vi "Resize.vi"(8 "error in (no error)":errorcluster, 10 "Pane.Content Area Rect":T1, 11 "Loop data in":T2 {"PanelMap"."Data"."Plot Bounds (%)"."Bottom (%)" format="%.2f"; "PanelMap"."Data"."Plot Bounds (%)"."Top (%)" format="%.2f"; "PanelMap"."Data"."Plot Bounds (%)"."Right (%)" format="%.2f"; "PanelMap"."Data"."Plot Bounds (%)"."Left (%)" format="%.2f"}) -> (0 "error out":errorcluster, 3 "Loop data out":T2 {"PanelMap"."Data"."Plot Bounds (%)"."Bottom (%)" format="%.2f"; "PanelMap"."Data"."Plot Bounds (%)"."Top (%)" format="%.2f"; "PanelMap"."Data"."Plot Bounds (%)"."Right (%)" format="%.2f"; "PanelMap"."Data"."Plot Bounds (%)"."Left (%)" format="%.2f"})   [LabVIEW 2021, in "MultiStokePlot.lvlib" / "MultiPlotPanel.lvclass"]
uses:
  Classes/MultiPlotPanel/MultiPlotPanel.lvclass
  Loop Data.ctl
  <vilib>/IlluminatedG/IG OOPanel/OOPanel/Manager/Manager.lvclass
  Panel Map.ctl
  Panel Map Data.ctl
  <userlib>/bjustice/RocketPlot/Classes/RocketPlotPanel/RocketPlotPanel.lvclass
  Window Position.ctl
  <vilib>/IlluminatedG/IG OOPanel/OOPanel/Panel/Panel Events.ctl
  <vilib>/IlluminatedG/IG OOPanel/OOPanel/Panel/Visbility Event Data.ctl
  <vilib>/IlluminatedG/IG OOPanel/OOPanel/Visibility State.ctl
  <vilib>/IlluminatedG/IG OOPanel/OOPanel/Close Reason.ctl
  <vilib>/Utility/miscctls.llb/LVRectTypeDef.ctl
  <vilib>/Utility/miscctls.llb/LVBoundsTypeDef.ctl
  <vilib>/Utility/miscctls.llb/LVPositionTypeDef.ctl
  <vilib>/IlluminatedG/IG OOPanel/OOPanel/OOPanel.lvlib
  <vilib>/IlluminatedG/IG OOPanel/OOPanel/Panel/Panel.lvclass
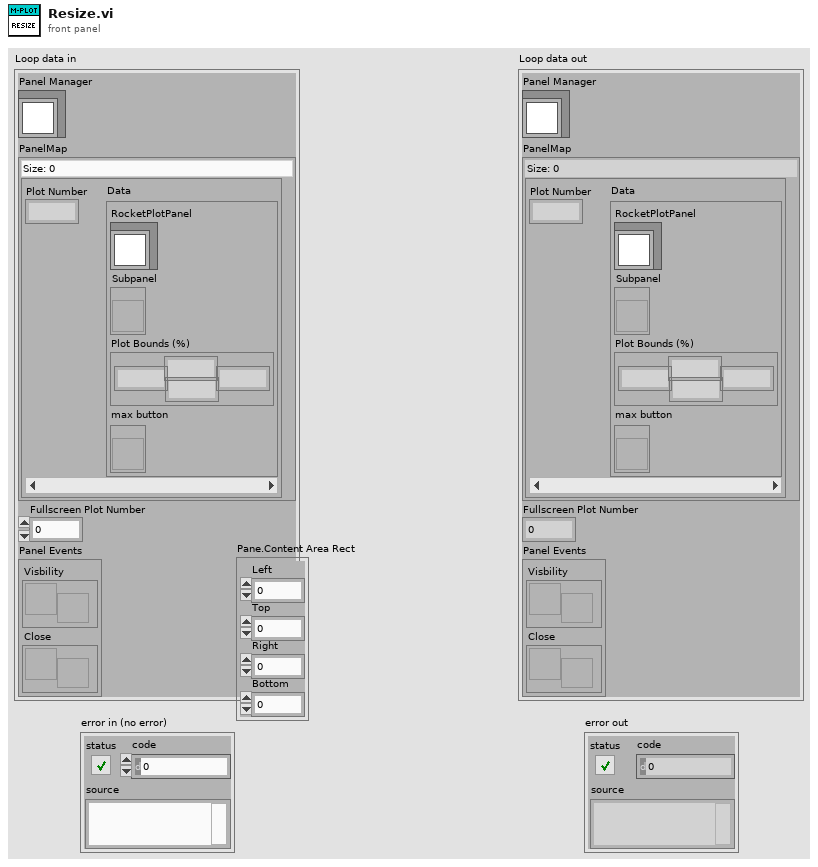
[diagram p1: front panel]
types:
  T1 = typedef "LVRectTypeDef.ctl" = cluster{"Left":i16, "Top":i16, "Right":i16, "Bottom":i16}
  T2 = typedef "MultiStokePlot.lvlib/MultiPlotPanel.lvclass/Loop Data.ctl" = cluster{"Panel Manager":refnum<class "Manager.lvclass">, "PanelMap":T3, "Fullscreen Plot Number":i32, "Panel Events":T6}
  T3 = typedef "MultiStokePlot.lvlib/MultiPlotPanel.lvclass/Panel Map.ctl" = map{i32, T4}
  T4 = typedef "MultiStokePlot.lvlib/MultiPlotPanel.lvclass/Panel Map Data.ctl" = cluster{"RocketPlotPanel":refnum<class "RocketPlotPanel.lvclass">, "Subpanel":refnum<vi>, "Plot Bounds (%)":T5, "max button":refnum<vi>}
  T5 = typedef "MultiStokePlot.lvlib/MultiPlotPanel.lvclass/Window Position.ctl" = cluster{"Left (%)":dbl, "Top (%)":dbl, "Right (%)":dbl, "Bottom (%)":dbl}
  T6 = typedef "OOPanel.lvlib/Panel.lvclass/Panel Events.ctl" = cluster{"Visbility":refnum<user-event>, "Close":refnum<user-event>}
  T7 = typedef "LVPositionTypeDef.ctl" = cluster{"Left":i32, "Top":i32}
  T8 = typedef "LVBoundsTypeDef.ctl" = cluster{"Width":u32, "Height":u32}
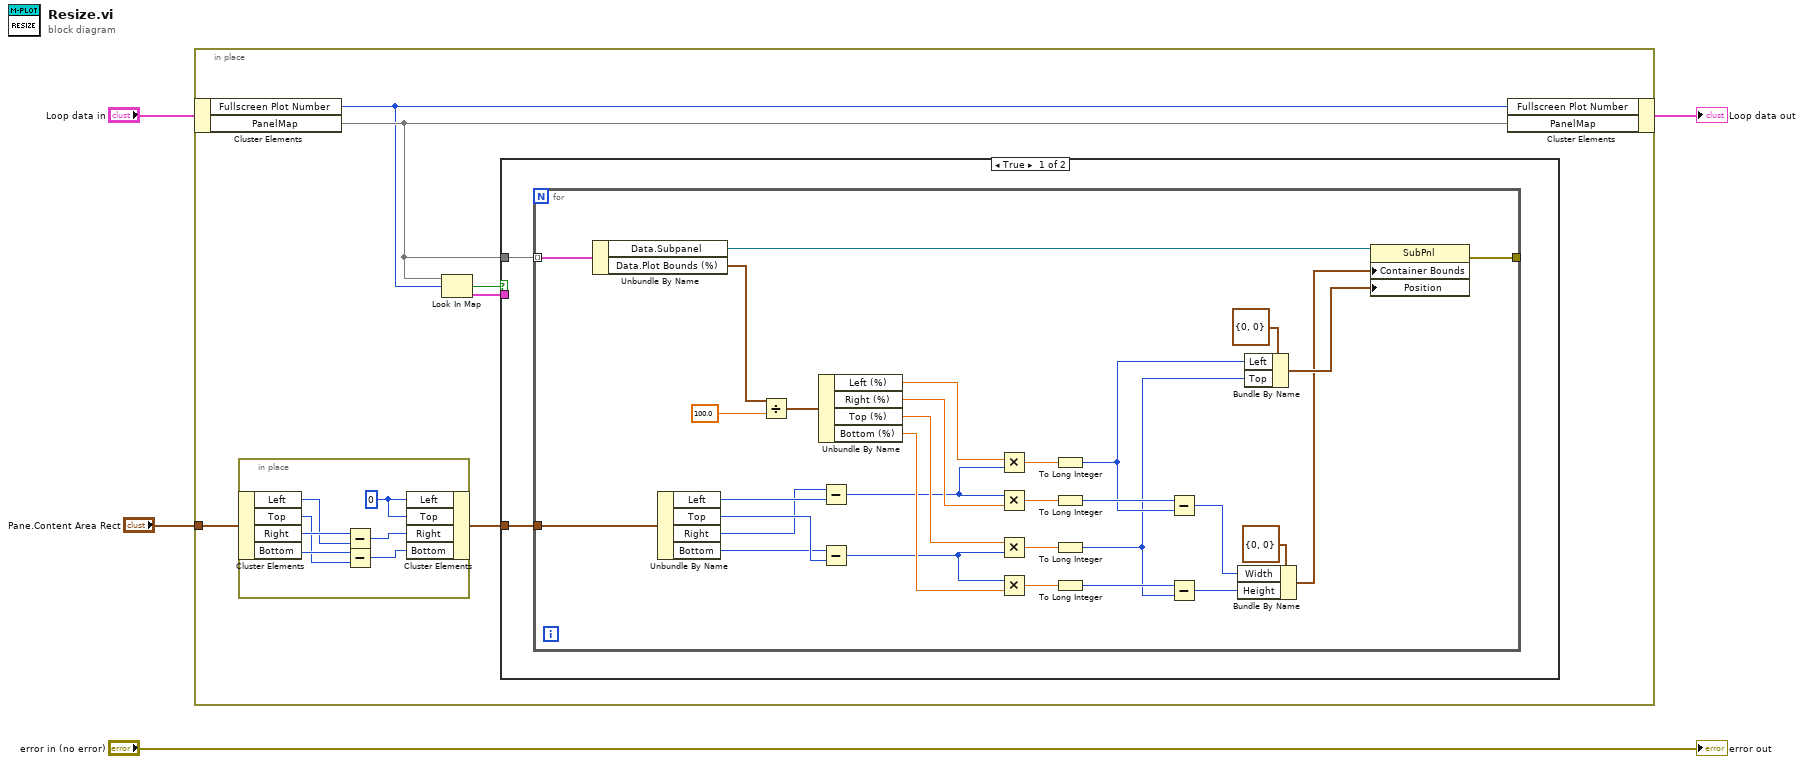
[diagram p0: block diagram]
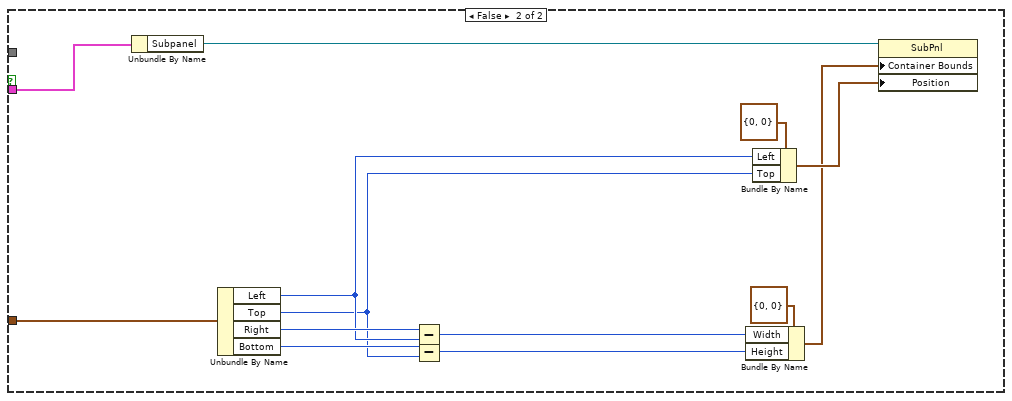
[diagram p2: hidden frame]
diagram:
  n1 = in-place {
    in-place-border: "Pane.Content Area Rect" -> [w6]
    n2 = in-place-cluster #1("Loop data in") -> ("Fullscreen Plot Number"=w9:i32, "PanelMap"=w10:T3)
    n3 = in-place {
      w17 = i16 0 ("Left")
      n4 = in-place-cluster #2(w6) -> ("Left"=w15:i16, "Top"=w12:i16, "Right"=w16:i16, "Bottom"=w13:i16)
      n5 = Subtract(x=w16, y=w15) -> (x-y=w14:i16)
      n6 = Subtract(x=w13, y=w12) -> (x-y=w11:i16)
      n7 = in-place-cluster #2("Left"=w17, "Top"=w17, "Right"=w14, "Bottom"=w11) -> (w5:T1)
    }
    n8 = Look In Map(map=w10, key=w9) -> (key not found?=w8:bool, value=w7:T4)  [unwired: 1 in]
    n9 = case shown="True" w8 {
      tunnel: w10 -> [w19 _]
      tunnel: w7 -> [_ w63]
      tunnel: w5 -> [w18 w62]
      frame True {
        n10 = for {
          tunnel: w19 -> [w50] mode=indexing
          tunnel: [w44] -> _
          tunnel: w18 -> [w22]
          n11 = Unbundle By Name(w50) -> ("Data.Subpanel"=w48:refnum<vi>, "Data.Plot Bounds (%)"=w37:T5)
          n12 = Unbundle By Name(w22) -> ("Left"=w24:i16, "Top"=w26:i16, "Right"=w23:i16, "Bottom"=w25:i16)
          n13 = Divide(x=w37, y=100.0 ("Right (%)")) -> (x/y=w42:T5)
          n14 = Unbundle By Name(w42) -> ("Left (%)"=w41:dbl, "Right (%)"=w39:dbl, "Top (%)"=w38:dbl, "Bottom (%)"=w40:dbl)
          n15 = Subtract(x=w23, y=w24) -> (x-y=w21:i16)
          n16 = Subtract(x=w25, y=w26) -> (x-y=w20:i16)
          n17 = Multiply(x=w41, y=w21) -> (x*y=w36:dbl)
          n18 = Multiply(x=w21, y=w39) -> (x*y=w35:dbl)
          n19 = Multiply(x=w38, y=w20) -> (x*y=w34:dbl)
          n20 = Multiply(x=w20, y=w40) -> (x*y=w33:dbl)
          n21 = To Long Integer(number=w36) -> (32bit integer=w31:i32)
          n22 = To Long Integer(number=w35) -> (32bit integer=w32:i32)
          n23 = To Long Integer(number=w34) -> (32bit integer=w28:i32)
          n24 = To Long Integer(number=w33) -> (32bit integer=w29:i32)
          n25 = Subtract(x=w32, y=w31) -> (x-y=w30:i32)
          n26 = Subtract(x=w29, y=w28) -> (x-y=w27:i32)
          n27 = Bundle By Name(cluster=T8 {"Width"=0, "Height"=0} ("Container Bounds"), "Width"=w30, "Height"=w27) -> (w45:T8)
          n28 = Bundle By Name(cluster=T7 {"Left"=0, "Top"=0} ("Position"), "Left"=w31, "Top"=w28) -> (w46:T7)
          n29 = property class="SubPnl"(reference=w48, "Container Bounds"=w45, "Position"=w46) -> (error out=w44:errorcluster)  [unwired: 1 in, 1 out]
        }
      }
      frame False {
        n30 = Unbundle By Name(w63) -> ("Subpanel"=w60:refnum<vi>)
        n31 = Unbundle By Name(w62) -> ("Left"=w55:i16, "Top"=w52:i16, "Right"=w56:i16, "Bottom"=w53:i16)
        n32 = Subtract(x=w56, y=w55) -> (x-y=w54:i16)
        n33 = Subtract(x=w53, y=w52) -> (x-y=w51:i16)
        n34 = Bundle By Name(cluster=T8 {"Width"=0, "Height"=0} ("Container Bounds"), "Width"=w54, "Height"=w51) -> (w57:T8)
        n35 = Bundle By Name(cluster=T7 {"Left"=0, "Top"=0} ("Position"), "Left"=w55, "Top"=w52) -> (w58:T7)
        n36 = property class="SubPnl"(reference=w60, "Container Bounds"=w57, "Position"=w58) -> ()  [unwired: 1 in, 2 out]
      }
    }
    n37 = in-place-cluster #1("Fullscreen Plot Number"=w9, "PanelMap"=w10) -> (→"Loop data out":T2)
  }
  "error out" <- "error in (no error)"
